vi "testA.vi"() -> ()   [LabVIEW 2016]
panel:
  in  "Start D":bool
  in  "OK D":bool
  in  "Stop D":bool
  in  "In B":i32
  out "Internal B":i32
  out "Internal C":i32
  in  "Stop C":bool
  out "Internal A":i32
  in  "Start B":bool
  in  "Bouton A":bool
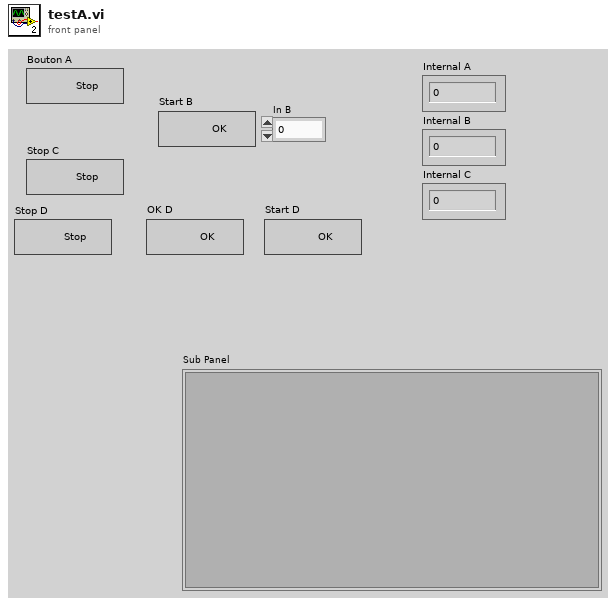
[diagram p1: front panel]
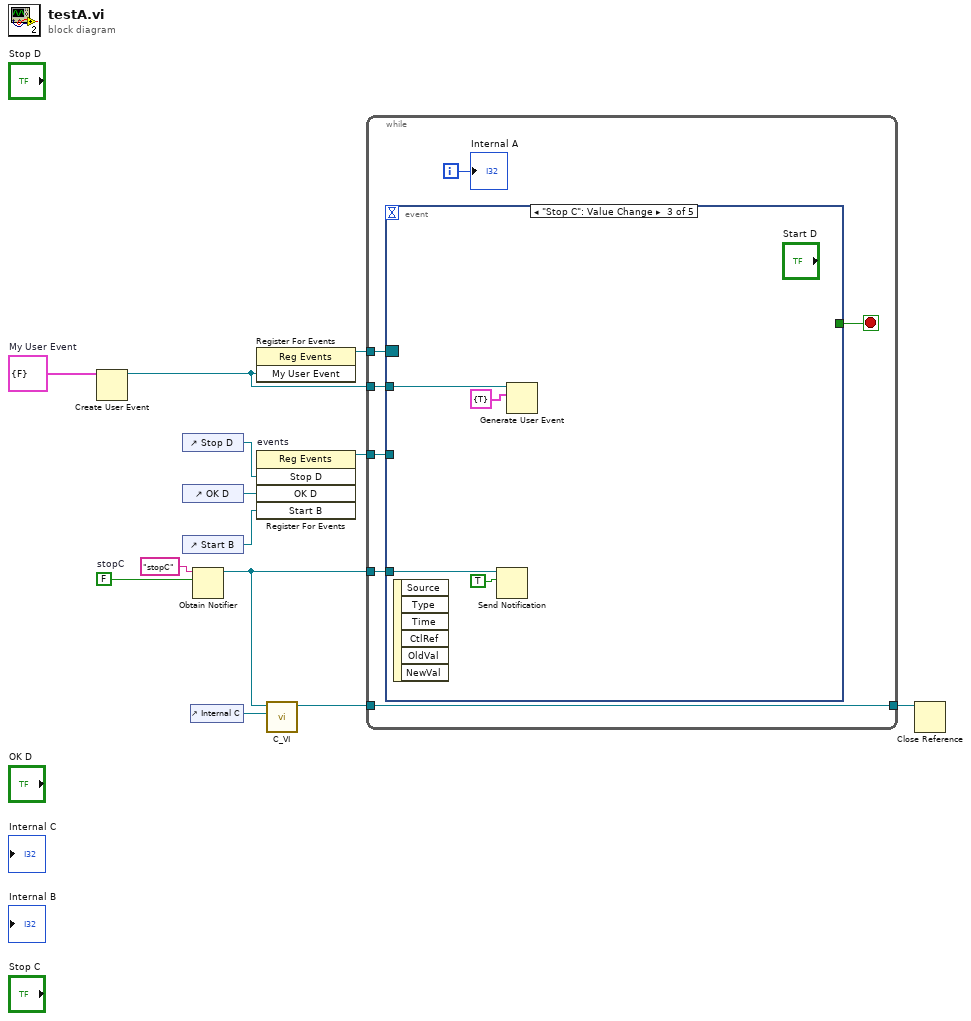
[diagram p0: block diagram]
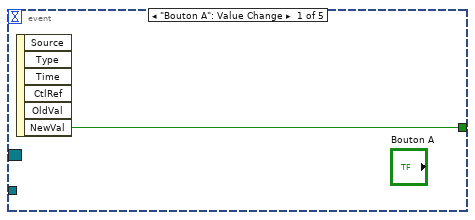
[diagram p2: hidden frame]
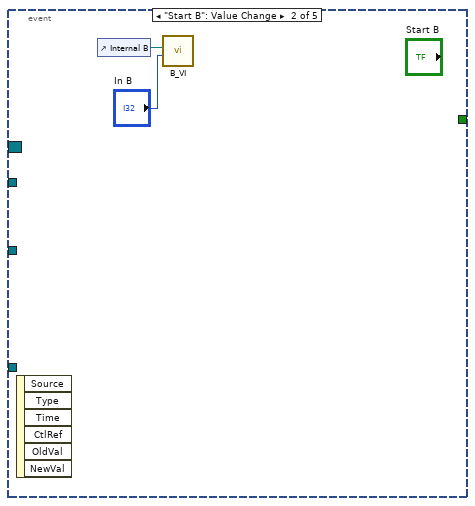
[diagram p3: hidden frame]
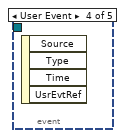
[diagram p4: hidden frame]
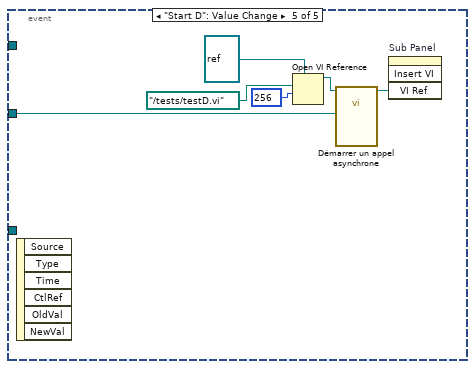
[diagram p5: hidden frame]
diagram:
  w9 = FALSE  # stopC
  w13 = cluster{"stopC":bool} {"stopC"=FALSE}  # My User Event
  n1 = Create User Event(user event datatype=w13) -> (user event=w11:refnum<user-event>)  [unwired: 1 in, 1 out]
  n2 = control-ref of="Stop D"() -> (w4:refnum<vi>)
  n3 = control-ref of="OK D"() -> (w3:refnum<vi>)
  n4 = control-ref of="Start B"() -> (w2:refnum<vi>)
  n5 = control-ref of="Internal C"() -> (w5:refnum<vi>)
  n6 = Obtain Notifier(name (unnamed)="stopC", notification data type=w9) -> (notifier out=w8:refnum<notifier>)  [unwired: 2 in, 2 out]
  n7 = register-events(w11) -> (reference out=w12:refnum<event-registration>)  [unwired: 2 in, 1 out]
  n8 = register-events "events"(w4, w3, w2) -> (reference out=w1:refnum<event-registration>)  [unwired: 2 in, 1 out]
  n9 = call "C_VI.vi"("Internal C"=w5, "Notifier in"=w8) -> ("VI out"=w7:refnum<vi>)  [unwired: 9 in]
  n10 = while {
    tunnel: w12 -> [w19]
    tunnel: w11 -> [w18]
    tunnel: w8 -> [w17]
    tunnel: [w16] -> w6
    tunnel: w7 -> [w16]
    tunnel: w1 -> [w14]
    i -> [w15]
    stop <- w20 stop-if-true
    n11 = event shown="[2] \"Stop C\": Value Change" {
      selector: w19 -> [_ _ _ _ _]
      dyn-events: _ -> [_ _ _ _ _]
      timeout: _ -> [_ _ _ _ _]
      tunnel: [w21 _ _ _ _] -> w20
      tunnel: w18 -> [_ _ w26 _ _]
      tunnel: w17 -> [_ _ w25 _ _]
      tunnel: w14 -> [_ _ _ _ w29]
      event "Bouton A": Value Change {
        n12 = event-data() -> ("NewVal"=w21:bool)  [unwired: 1 in, 5 out]
      }
      event "Start B": Value Change {
        n13 = event-data() -> ()  [unwired: 1 in, 6 out]
        n14 = control-ref of="Internal B"() -> (w22:refnum<vi>)
        n15 = call "B_VI.vi"("In B"="In B", "Internal B"=w22) -> ()  [unwired: 10 in]
      }
      event "Stop C": Value Change {
        n16 = event-data() -> ()  [unwired: 1 in, 6 out]
        n17 = Send Notification(notification=TRUE, notifier=w25) -> ()  [unwired: 1 in, 2 out]
        n18 = Generate User Event(user event=w26, event data cluster=cluster{bool} {TRUE} ("event data")) -> ()  [unwired: 2 in, 2 out]
      }
      event User Event {
        n19 = event-data() -> ()  [unwired: 1 in, 4 out]
      }
      event "Start D": Value Change {
        n20 = event-data() -> ()  [unwired: 1 in, 6 out]
        n21 = Open VI Reference(type specifier VI Refnum (for type only)=refnum<vi> refnum ("spécificateur de type du refnum de VI (pour type seulement)"), vi path=path "../tests/testD.vi" ("chemin du VI"), options=256) -> (vi reference=w33:refnum<vi>)  [unwired: 3 in, 1 out]
        n22 = call-by-ref "Démarrer un appel asynchrone"(reference=w33, "Event Registration Refnum"=w29) -> (reference out=w28:refnum<vi>)  [unwired: 12 in, 1 out]
        n23 = invoke on="Sub Panel" class="SubPnl" method="Insert VI"("VI Ref"=w28) -> ()  [unwired: 3 in, 4 out]
      }
    }
    "Internal A" <- w15
  }
  n24 = Close Reference(reference=w6) -> ()  [unwired: 1 in, 1 out]
